vi "读取配置.vi"(7 "refnum":T4 caption="引用句柄", 10 "测试人员":string, 11 "错误输入（无错误）":errorcluster) -> (0 "脉冲":T2 {"测试参数"."反向极限电流(mA)" min=0.0 max=3000.0; "测试参数"."反向电压(V)" min=0.0 max=40.0; "测试参数"."读取电压(V)" min=0.0 max=40.0; "测试参数"."正向极限电流(mA)" min=0.0 max=3000.0; "测试参数"."正向电压(V)" min=0.0 max=40.0}, 1 "维持时间":T1={"测试参数"={"读取电压(V)"=0.0, "极限电流(mA)"=0.0}, "时序参数"={"测试时间(s)"=0.0, "读取间隔(ms)"=0.0, "nplc"=0.001, "时序优先"=FALSE}} {"时序参数"."nplc" min=0.001; "测试参数"."极限电流(mA)" min=0.0 max=3000.0; "测试参数"."读取电压(V)" min=0.0 max=40.0}, 3 "错误输出":errorcluster, 4 "扫描":T3={"测试参数"={"正向电压(V)"=0.0, "正向极限电流(mA)"=0.0, "反向电压(V)"=0.0, "反向极限电流(mA)"=0.0, "电压改变量(V)"=0.0}, "时序参数"={"维持时间(ms)"=0.0, "nplc"=0.001, "时序优先"=FALSE}} {"测试参数"."反向极限电流(mA)" min=0.0 max=3000.0; "测试参数"."反向电压(V)" min=0.0 max=40.0; "测试参数"."电压改变量(V)" min=0.0 max=40.0 step=5e-06; "测试参数"."正向极限电流(mA)" min=0.0 max=3000.0; "测试参数"."正向电压(V)" min=0.0 max=40.0; "时序参数"."nplc" min=0.001}, 5 "refnum out":T4 caption="引用句柄输出", 6 "样品标记":string[](array[string]))   [LabVIEW 2021]
uses:
  <vilib>/Utility/config.llb/Config Data RefNum.ctl
  <vilib>/Utility/config.llb/Read Key (String).vi
  <vilib>/Utility/config.llb/NI_LVConfig.lvlib
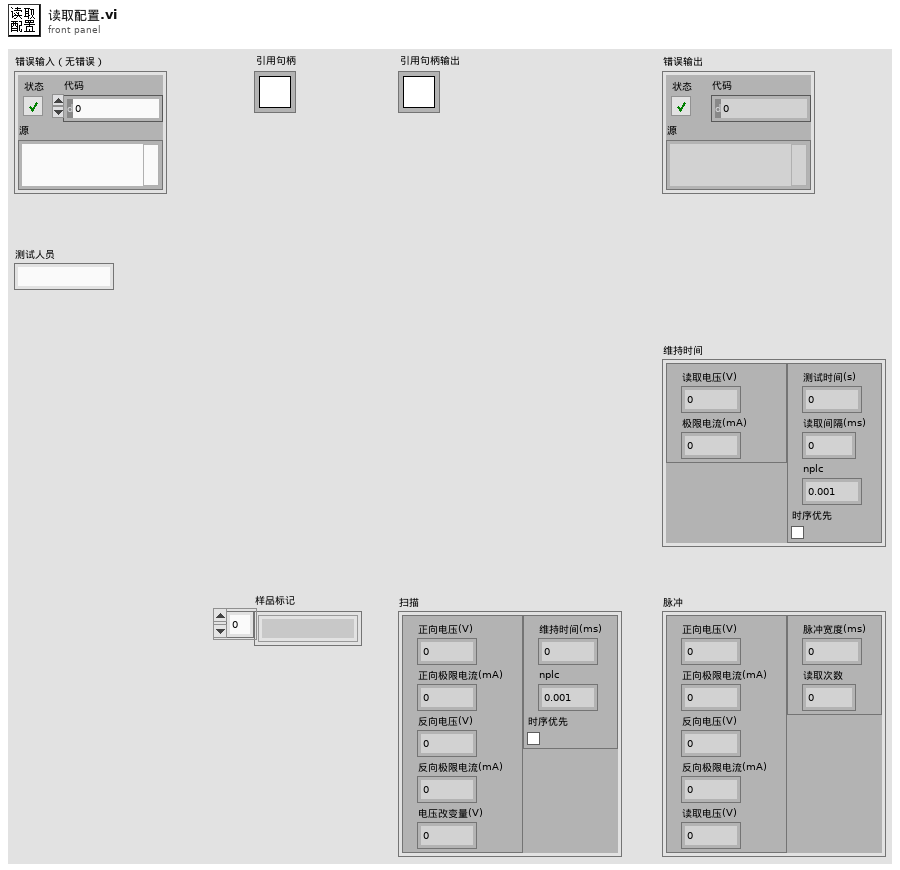
[diagram p1: front panel]
types:
  T1 = typedef "维持时间.ctl" = cluster{"测试参数":cluster{"读取电压(V)":dbl, "极限电流(mA)":dbl}, "时序参数":cluster{"测试时间(s)":dbl, "读取间隔(ms)":dbl, "nplc":dbl, "时序优先":bool}}
  T2 = typedef "脉冲参数.ctl" = cluster{"测试参数":cluster{"正向电压(V)":dbl, "正向极限电流(mA)":dbl, "反向电压(V)":dbl, "反向极限电流(mA)":dbl, "读取电压(V)":dbl}, "时序参数":cluster{"脉冲宽度(ms)":dbl, "读取次数":u32}}
  T3 = typedef "扫描参数.ctl" = cluster{"测试参数":cluster{"正向电压(V)":dbl, "正向极限电流(mA)":dbl, "反向电压(V)":dbl, "反向极限电流(mA)":dbl, "电压改变量(V)":dbl}, "时序参数":cluster{"维持时间(ms)":dbl, "nplc":dbl, "时序优先":bool}}
  T4 = typedef "NI_LVConfig.lvlib/Config Data RefNum.ctl" = refnum<k1>
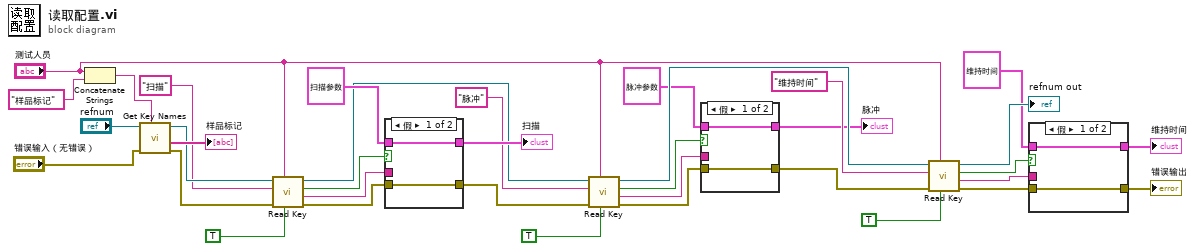
[diagram p0: block diagram]
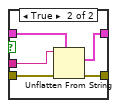
[diagram p2: hidden frame]
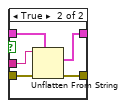
[diagram p3: hidden frame]
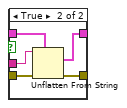
[diagram p4: hidden frame]
diagram:
  n1 = Concatenate Strings("测试人员", "样品标记" ("字符串")) -> (w34:string)
  n2 = call <vilib>:"Get Key Names.vi"("section"=w34, "error in (no error)"="错误输入（无错误）", "refnum"="refnum") -> ("error out"=w27:errorcluster, "key names"=→"样品标记":string[], "refnum out"=w30:T4)  [unwired: 5 in, 1 out]
  n3 = call-poly <vilib>:"Read Key.vi"("read raw string? (F)"=TRUE, "section"="测试人员", "error in (no error)"=w27, "key"="扫描", "refnum"=w30) -> ("error out"=w7:errorcluster, "value"=w25:string, "found?"=w26:bool, "refnum out"=w21:T4)  [unwired: 3 in]
  n4 = case shown="假" w26 {
    tunnel: w25 -> [_ w42]
    tunnel: T3 {"测试参数"={"正向电压(V)"=1.0, "正向极限电流(mA)"=1.0, "反向电压(V)"=1.0, "反向极限电流(mA)"=1.0, "电压改变量(V)"=0.1}, "时序参数"={"维持时间(ms)"=25.0, "nplc"=0.1, "时序优先"=FALSE}} ("扫描") -> [w37 w41]
    tunnel: [w37 w40] -> w23
    tunnel: [w36 w39] -> w6
    tunnel: w7 -> [w36 w38]
    frame False {
    }
    frame True {
      n5 = Unflatten From String(type=w41, binary string=w42, error in (no error)=w38) -> (value=w40:T3, error out=w39:errorcluster)  [unwired: 2 in, 1 out]
    }
  }
  "扫描" <- w23
  n6 = call-poly <vilib>:"Read Key.vi"("read raw string? (F)"=TRUE, "section"="测试人员", "error in (no error)"=w6, "key"="脉冲", "refnum"=w21) -> ("error out"=w5:errorcluster, "value"=w15:string, "found?"=w16:bool, "refnum out"=w19:T4)  [unwired: 3 in]
  n7 = case shown="假" w16 {
    tunnel: w15 -> [_ w49]
    tunnel: T2 {"测试参数"={"正向电压(V)"=1.0, "正向极限电流(mA)"=1.0, "反向电压(V)"=1.0, "反向极限电流(mA)"=1.0, "读取电压(V)"=0.1}, "时序参数"={"脉冲宽度(ms)"=20.0, "读取次数"=20}} ("脉冲") -> [w44 w48]
    tunnel: [w44 w47] -> w13
    tunnel: [w43 w46] -> w4
    tunnel: w5 -> [w43 w45]
    frame False {
    }
    frame True {
      n8 = Unflatten From String(type=w48, binary string=w49, error in (no error)=w45) -> (value=w47:T2, error out=w46:errorcluster)  [unwired: 2 in, 1 out]
    }
  }
  "脉冲" <- w13
  n9 = call-poly <vilib>:"Read Key.vi"("read raw string? (F)"=TRUE, "section"="测试人员", "error in (no error)"=w4, "key"="维持时间", "refnum"=w19) -> ("error out"=w3:errorcluster, "value"=w12:string, "found?"=w11:bool, "refnum out"=→"refnum out":T4)  [unwired: 3 in]
  n10 = case shown="假" w11 {
    tunnel: w12 -> [_ w56]
    tunnel: T1 {"测试参数"={"读取电压(V)"=1.0, "极限电流(mA)"=1.0}, "时序参数"={"测试时间(s)"=10.0, "读取间隔(ms)"=10.0, "nplc"=1.0, "时序优先"=FALSE}} ("维持时间") -> [w51 w55]
    tunnel: [w51 w54] -> w9
    tunnel: [w50 w53] -> w8
    tunnel: w3 -> [w50 w52]
    frame False {
    }
    frame True {
      n11 = Unflatten From String(type=w55, binary string=w56, error in (no error)=w52) -> (value=w54:T1, error out=w53:errorcluster)  [unwired: 2 in, 1 out]
    }
  }
  "错误输出" <- w8
  "维持时间" <- w9
